vi "Read Waveform.vi"(0 "RedPitaya TCP Connection in":refnum<k5>, 5 "error in":errorcluster, 6 "Channel #":u16(ring)=1 items=["Channel 1"=1, "Channel 2"=2], 12 "timeout ms (2000)":i32=2000) -> (14 "RedPitaya TCP Connection out":refnum<k5>, 16 "Measurement Array":dbl[](array[numeric]), 19 "error out":errorcluster)   [LabVIEW 2010, in "RedPitaya.lvlib"]
doc: "Read full buf. size starting from oldest sample in buffer (this is first sample after trigger delay). Trigger delay by default is set to zero (in samples or in seconds). If trigger delay is set to zero it will read full buf. size starting from trigger."
uses:
  RedPitaya.lvlib
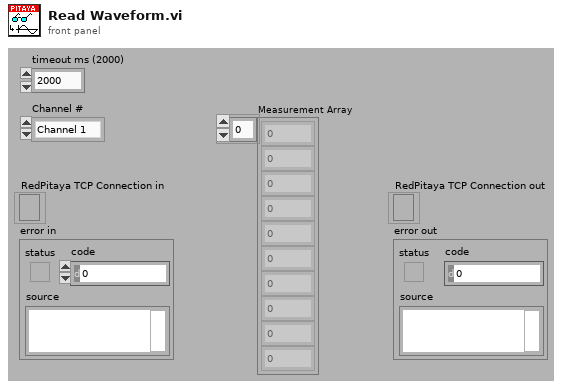
[diagram p1: front panel]
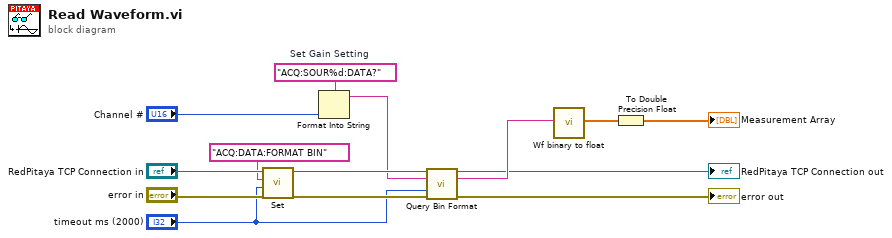
[diagram p0: block diagram]
diagram:
  w14 = "ACQ:SOUR%d:DATA?"  # Set Gain Setting
  n1 = call "Set.vi"("error in"="error in", "timeout ms (2000)"="timeout ms (2000)", "SCPI Message"="ACQ:DATA:FORMAT BIN", "RedPitaya connection in"="RedPitaya TCP Connection in") -> ("error out"=w7:errorcluster, "RedPitaya connection out"=w9:refnum<k5>)  [unwired: 5 in, 1 out]
  n2 = Format Into String(format string=w14, "Channel #") -> (resulting string=w8:string)  [unwired: 2 in, 1 out]
  n3 = call "Query Bin Format.vi"("RedPitaya connection in"=w9, "SCPI Query"=w8, "timeout ms (2000)"="timeout ms (2000)", "error in"=w7) -> ("RedPitaya connection out"=→"RedPitaya TCP Connection out":refnum<k5>, "data out"=w6:string, "error out"=→"error out":errorcluster)  [unwired: 9 in]
  n4 = call "Wf binary to float.vi"("Input string"=w6) -> ("Data out"=w2:sgl[])  [unwired: 18 in]
  n5 = To Double Precision Float(number=w2) -> (double precision float=→"Measurement Array":dbl[])
